vi "ZBX IO DB.vi"(7 "DBoard IOs":T1={"CtrlPortReqAddr"="Daughterboard 0\\DBoardCtrlPortReqAddr", "CtrlPortReqData"="Daughterboard 0\\DBoardCtrlPortReqData", "CtrlPortReqWr"="Daughterboard 0\\DBoardCtrlPortReqWr", "CtrlPortReqRd"="Daughterboard 0\\DBoardCtrlPortReqRd", "CtrlPortReqHasTime"="Daughterboard 0\\DBoardCtrlPortReqHasTime", "CtrlPortReqTime"="Daughterboard 0\\DBoardCtrlPortReqTime", "CtrlPortRespAck"="Daughterboard 0\\DBoardCtrlPortRespAck", "CtrlPortRespData"="Daughterboard 0\\DBoardCtrlPortRespData", "CtrlPortRespStatus"="Daughterboard 0\\DBoardCtrlPortRespStatus"}, 11 "request":T3) -> (3 "response":T2)   [LabVIEW 2023]
doc: "Does the actual IO for requests/responses to daugtherbord 0.\nNote: Put only <strong>one>/strong> instance of this VI in your FPGA. When multiple requests are send to the daugtherboard use the arbiter VI."
uses:
  <vilib>/eio/EIONode/EIONode.xnode
  <instrlib>/niUSRP/Reference FPGA/ZBX Control/ZBX IO Response.ctl
  <vilib>/rvi/eio/common/nirviEmuTemplateMethod_errors.vi
  <instrlib>/niUSRP/Reference FPGA/ZBX Control/ZBX IO Request.ctl
  <instrlib>/niUSRP/Reference FPGA/ZBX Control/Dboard IOs.ctl
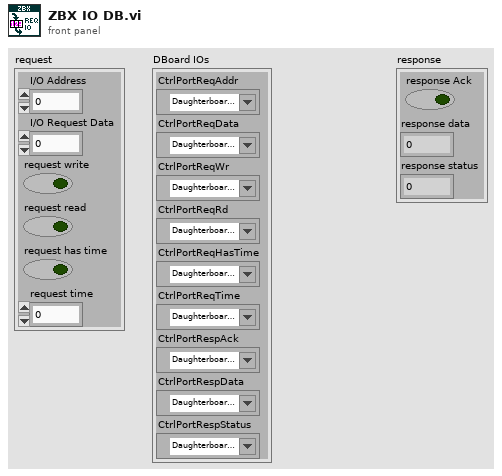
[diagram p1: front panel]
types:
  T1 = typedef "Dboard IOs.ctl" = cluster{"CtrlPortReqAddr":refnum<k21>, "CtrlPortReqData":refnum<k21>, "CtrlPortReqWr":refnum<k21>, "CtrlPortReqRd":refnum<k21>, "CtrlPortReqHasTime":refnum<k21>, "CtrlPortReqTime":refnum<k21>, "CtrlPortRespAck":refnum<k21>, "CtrlPortRespData":refnum<k21>, "CtrlPortRespStatus":refnum<k21>}
  T2 = typedef "ZBX IO Response.ctl" = cluster{"response Ack":bool, "response data":u32, "response status":fxp<+,2,2>}
  T3 = typedef "ZBX IO Request.ctl" = cluster{"I/O Address":fxp<+,20,20>, "I/O Request Data":u32, "request write":bool, "request read":bool, "request has time":bool, "request time":u64}
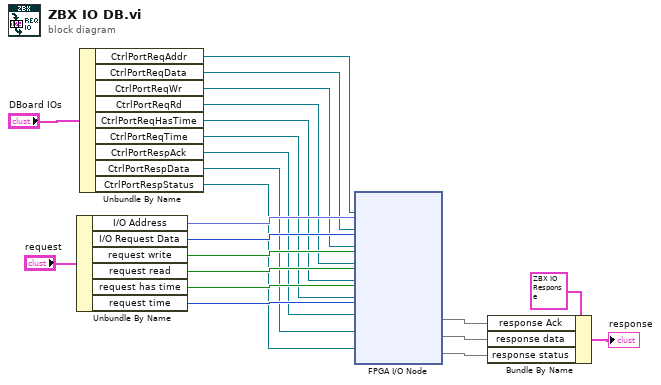
[diagram p0: block diagram]
diagram:
  n1 = Unbundle By Name("request") -> ("I/O Address"=w22:fxp<+,20,20>, "I/O Request Data"=w21:u32, "request write"=w20:bool, "request read"=w19:bool, "request has time"=w18:bool, "request time"=w17:u64)
  n2 = Unbundle By Name("DBoard IOs") -> ("CtrlPortReqAddr"=w9:refnum<k21>, "CtrlPortReqData"=w8:refnum<k21>, "CtrlPortReqWr"=w7:refnum<k21>, "CtrlPortReqRd"=w6:refnum<k21>, "CtrlPortReqHasTime"=w5:refnum<k21>, "CtrlPortReqTime"=w4:refnum<k21>, "CtrlPortRespAck"=w3:refnum<k21>, "CtrlPortRespData"=w2:refnum<k21>, "CtrlPortRespStatus"=w1:refnum<k21>)
  n3 = xnode "FPGA I/O Node"("I/O Item"=w22, "FPGA I/O In"=w9, "I/O Item"=w21, "FPGA I/O In"=w8, "I/O Item"=w20, "FPGA I/O In"=w7, "I/O Item"=w19, "FPGA I/O In"=w6, "I/O Item"=w18, "FPGA I/O In"=w5, "I/O Item"=w17, "FPGA I/O In"=w4, "FPGA I/O In"=w3, "FPGA I/O In"=w2, "FPGA I/O In"=w1) -> ("I/O Item"=w13, "I/O Item"=w12, "I/O Item"=w11)  [unwired: 9 out]
  n4 = Bundle By Name(cluster=T2 {"response Ack"=FALSE, "response data"=0, "response status"=0.0} ("Cluster"), "response Ack"=w13, "response data"=w12, "response status"=w11) -> (→"response":T2)
